vi "SD-Compare Two Paths.vi"(8 "error in (no error)":errorcluster, 10 "Path 2":path, 11 "Path 1":path) -> (0 "error out":errorcluster, 1 "Path 2 Relative to Path 1?":bool, 2 "Common Path":path, 3 "Relative Path from 1 to 2":path)   [LabVIEW 2020]
doc: "Compares<B> Path 1</B> to <B>Path 2</B> and returns a relative path between the two paths, the common path between the two paths, and a Boolean that indicates whether the paths are on the same path hierarchy level."
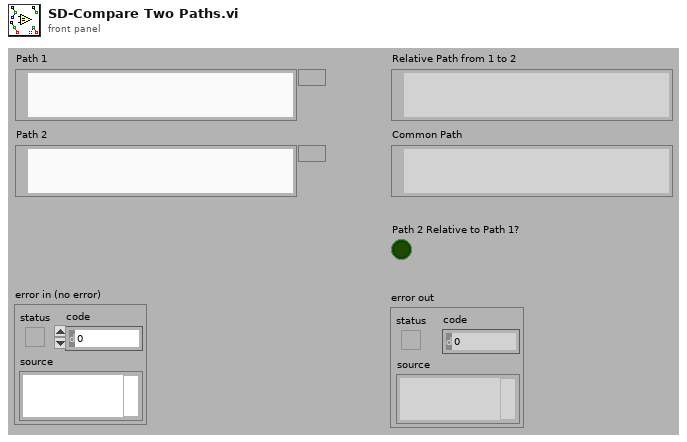
[diagram p1: front panel]
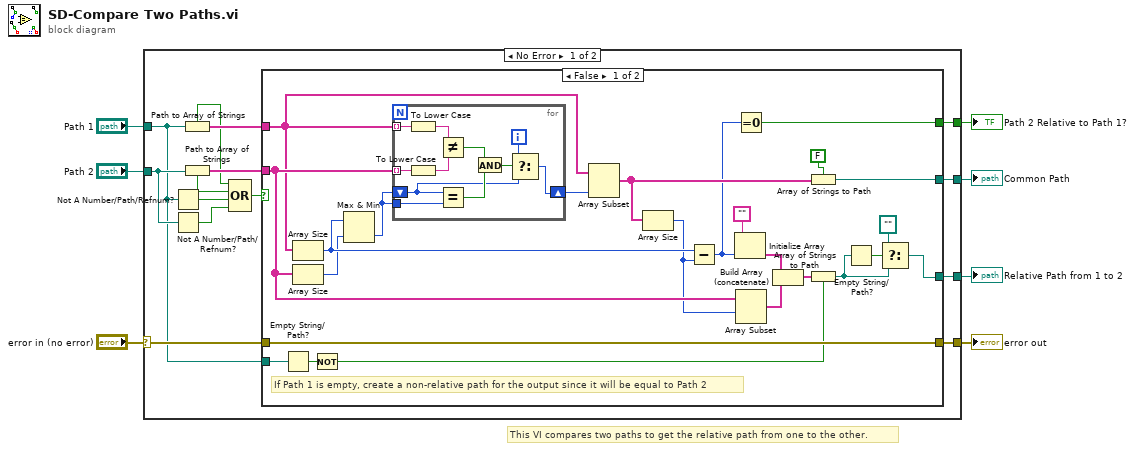
[diagram p0: block diagram]
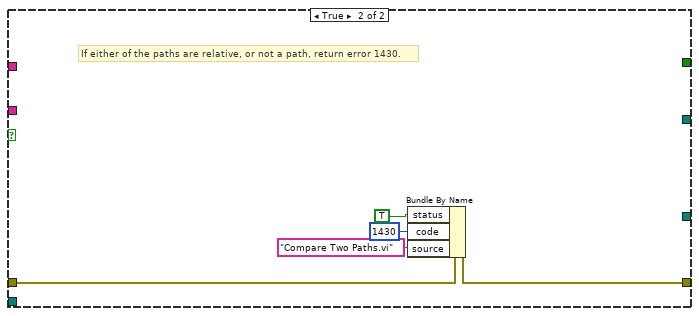
[diagram p2: hidden frame]
diagram:
  # "This VI compares two paths to get the relative path from one to the other."
  n1 = case shown="No Error" "error in (no error)" {
    selector: "error in (no error)" -> [w16 w62]
    tunnel: "Path 1" -> [w8 _]
    tunnel: "Path 2" -> [w9 _]
    tunnel: [w19 _] -> w5
    tunnel: [w18 _] -> w4
    tunnel: [w17 _] -> w3
    tunnel: [w15 w62] -> w1
    frame No Error {
      n2 = Not A Number/Path/Refnum?(number/path/refnum=w8) -> (NaN/Path/Refnum?=w11:bool)
      n3 = Not A Number/Path/Refnum?(number/path/refnum=w9) -> (NaN/Path/Refnum?=w10:bool)
      n4 = Path to Array of Strings(0:w8) -> (1:w12:bool, 2:w21:string[])
      n5 = Path to Array of Strings(0:w9) -> (1:w13:bool, 2:w20:string[])
      n6 = Compound Arithmetic op=OR(w12, w13, w11, w10) -> (w14:bool)
      n7 = case shown="False" w14 {
        tunnel: w21 -> [w37 _]
        tunnel: w20 -> [w40 _]
        tunnel: [w43 _] -> w19
        tunnel: [w23 _] -> w18
        tunnel: [w31 _] -> w17
        tunnel: w16 -> [w29 w61]
        tunnel: [w29 w60] -> w15
        tunnel: w8 -> [w28 _]
        frame False {
          # "If Path 1 is empty, create a non-relative path for the output since it will be equal to Path 2"
          n8 = Empty String/Path?(string/path=w28) -> (empty?=w27:bool)
          n9 = Array Size(array=w37) -> (size(s)=w36:i32)
          n10 = Array Size(array=w40) -> (size(s)=w35:i32)
          n11 = Not(x=w27) -> (.not. x?=w26:bool)
          n12 = Max & Min(x=w36, y=w35) -> (min(x,y)=w34:i32)  [unwired: 1 out]
          n13 = for {
            tunnel: w37 -> [w56] mode=indexing
            tunnel: w40 -> [w55] mode=indexing
            shift-right: [w48] -> w45
            shift-left: w34 -> [w49]
            tunnel: w34 -> [w54]
            i -> [w50]
            n14 = To Lower Case(string=w56) -> (all lower case string=w47:string)
            n15 = To Lower Case(string=w55) -> (all lower case string=w46:string)
            n16 = Not Equal?(x=w47, y=w46) -> (x != y?=w52:bool)
            n17 = Equal?(x=w49, y=w54) -> (x = y?=w53:bool)
            n18 = And(x=w52, y=w53) -> (x .and. y?=w51:bool)
            n19 = Select(t=w50, s=w51, f=w49) -> (s? t:f=w48:i32)
          }
          n20 = Array Subset(array=w37, length=w45) -> (w42:string[])  [unwired: 1 in]
          n21 = Array Size(array=w42) -> (size(s)=w33:i32)
          n22 = Subtract(x=w36, y=w33) -> (x-y=w32:i32)
          n23 = Initialize Array("", w32) -> (w41:string[])
          n24 = Equal To 0?(x=w32) -> (x = 0?=w31:bool)
          n25 = Array Subset(array=w40, index=w33) -> (w39:string[])  [unwired: 1 in]
          n26 = Build Array (concatenate)(w41, w39) -> (w38:string[])
          n27 = Array of Strings to Path(0:w42, 1:FALSE ("relative")) -> (2:w43:path)
          n28 = Array of Strings to Path(0:w38, 1:w26) -> (2:w24:path)
          n29 = Empty String/Path?(string/path=w24) -> (empty?=w25:bool)
          n30 = Select(t=path "", s=w25, f=w24) -> (s? t:f=w23:path)
        }
        frame True {
          # "If either of the paths are relative, or not a path, return error 1430."
          n31 = Bundle By Name(cluster=w61, "status"=TRUE, "code"=1430, "source"="Compare Two Paths.vi") -> (w60:errorcluster)
        }
      }
    }
    frame Error {
    }
  }
  "Relative Path from 1 to 2" <- w4
  "Path 2 Relative to Path 1?" <- w3
  "Common Path" <- w5
  "error out" <- w1
